vi "Set Mode.vi"(0 "reference in":refnum<class "Simulated-PowerModule.lvclass">, 5 "mode":string, 11 "Error In":errorcluster) -> (4 "reference out":refnum<class "Simulated-PowerModule.lvclass">, 15 "Error Out":errorcluster)   [LabVIEW 2023, in "Simulated-PowerModule.lvlib" / "Simulated-PowerModule.lvclass"]
uses:
  Simulated-PowerModule.lvclass
  Simulated-PowerModule.lvclass/Simulated-PowerModule.ctl
  <vilib>/addons/_JKI.lib/Serialization/JSON/JKI JSON Serialization.lvlib
  Mode.ctl
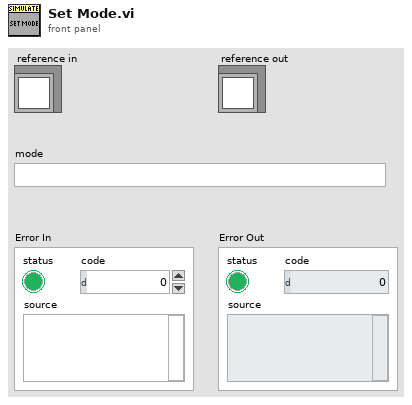
[diagram p1: front panel]
types:
  T1 = typedef "Simulated-PowerModule.lvlib/Simulated-PowerModule.lvclass/Mode.ctl" = u16
  T2 = typedef "Simulated-PowerModule.lvlib/Simulated-PowerModule.lvclass/ObjectAttributes.ctl" = cluster{"JSON Config Path":path, "Configuration":T3, "connected":bool, "reserved":bool, "energized":bool, "output enabled":bool, "Mode":T1, "Range":T4, "Slew Rates":T5, "Setpoints":cluster{"voltage":dbl, "current":dbl, "resistance":dbl}, "Measurements":cluster{"voltage":dbl, "current":dbl, "resistance":dbl}, "Limits":T6, "active faults":string[], "fault":bool}
  T3 = typedef "Simulated-PowerModule.lvlib/Simulated-PowerModule.lvclass/Configuration.ctl" = cluster{"IP Address":string}
  T4 = typedef "PowerModuleInterface.lvlibp/PowerModuleInterface.lvclass/Range.ctl" = cluster{"Current Max (A)":dbl, "Current Min (A)":dbl, "Voltage Max (V)":dbl, "Voltage Min (V)":dbl}
  T5 = typedef "PowerModuleInterface.lvlibp/PowerModuleInterface.lvclass/Slew Rates.ctl" = cluster{"Current Decrease (A/sec)":dbl, "Current Increase (A/sec)":dbl, "Voltage Decrease (V/sec)":dbl, "Voltage Increase (V/sec)":dbl, "Resistance Decrease (Ohm/sec)":dbl, "Resistance Increase (Ohm/sec)":dbl}
  T6 = typedef "PowerModuleInterface.lvlibp/PowerModuleInterface.lvclass/Limits.ctl" = cluster{"Current Max (A)":dbl, "Current Min (A)":dbl, "Voltage Max (V)":dbl, "Voltage Min (V)":dbl, "Power Max (W)":dbl, "Power Min (W)":dbl}
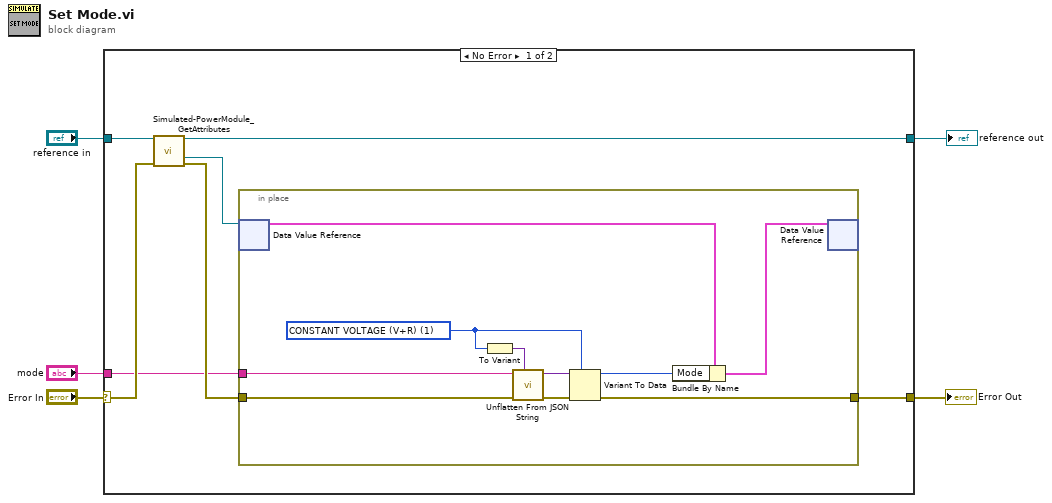
[diagram p0: block diagram]
diagram:
  n1 = case shown="No Error" "Error In" {
    selector: "Error In" -> [w11 w23]
    tunnel: "reference in" -> [w12 w24]
    tunnel: [w7 w24] -> w4
    tunnel: [w8 w23] -> w3
    tunnel: "mode" -> [w6 _]
    frame No Error {
      n2 = call "Simulated-PowerModule_GetAttributes.vi"("reference in"=w12, "Error In"=w11) -> ("reference out"=w7:refnum<class "Simulated-PowerModule.lvclass">, "DataRef"=w10:refnum<data-value>, "Error Out"=w9:errorcluster)  [unwired: 10 in, 1 out]
      n3 = in-place {
        in-place-border: w9 -> [w20]
        in-place-border: [w13] -> w8
        in-place-border: w6 -> [w19]
        w14 = T1 1 items=["CONSTANT VOLTAGE (V+R)"=1, "CONSTANT CURRENT (I)"=2] ("MODE")
        n4 = in-place-dvr #1(w10) -> (w21:T2)  [unwired: 1 out]
        n5 = To Variant(anything=w14) -> (Variant=w18:variant)
        n6 = call <vilib>:"Unflatten From JSON String.vi"("Type and Defaults"=w18, "error in"=w20, "JSON String"=w19) -> ("error out"=w17:errorcluster, "Variant"=w16:variant)  [unwired: 7 in]
        n7 = Variant To Data(error in=w17, type=w14, Variant=w16) -> (data=w15:T1, error out=w13:errorcluster)
        n8 = Bundle By Name(cluster=w21, "Mode"=w15) -> (w22:T2)
        n9 = in-place-dvr #1(w22) -> ()  [unwired: 2 out]
      }
    }
    frame Error {
    }
  }
  "Error Out" <- w3
  "reference out" <- w4
